vi "Init Tube Valves.vi"() -> (0 "Error Out":errorcluster, 2 "task out":refnum<k21>)   [LabVIEW 2016]
uses:
  <vilib>/DAQmx/create/channels.llb/DAQmx Create Channel (DO-Digital Output).vi
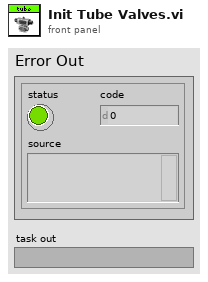
[diagram p1: front panel]
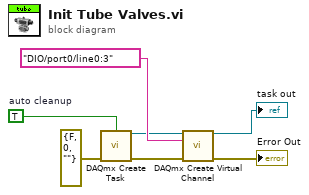
[diagram p0: block diagram]
diagram:
  w6 = TRUE  # auto cleanup
  n1 = call <vilib>:"DAQmx Create Task.vi"("auto cleanup"=w6, "error in"=errorcluster {"status"=FALSE, "code"=0, "source"=""}) -> ("task out"=w4:refnum<k21>, "error out"=w3:errorcluster)  [unwired: 12 in]
  n2 = call-poly <vilib>:"DAQmx Create Virtual Channel.vi"("task in"=w4, "lines"=tag "DIO/port0/line0:3", "error in"=w3) -> ("task out"=→"task out":refnum<k21>, "error out"=→"Error Out":errorcluster)  [unwired: 11 in]
